vi "Read Fan Status.vi"(11 "Update Fan Status Msg in":refnum<class "Update Fan Status Msg.lvclass">) -> (1 "Fan B":T1, 2 "Fan A":T1)   [LabVIEW 2018, in "Dual Fan.lvlib" / "Update Fan Status Msg.lvclass"]
doc: "Reads the fan status recorded in this message."
uses:
  Update Fan Status Msg.lvclass
  Dual Fan/Fan Info.ctl
  Update Fan Status Msg.lvclass/Update Fan Status Msg.ctl
  Dual Fan/Dual Fan.lvclass
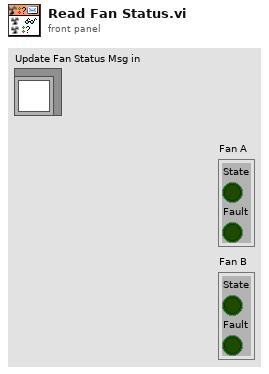
[diagram p1: front panel]
types:
  T1 = typedef "Dual Fan.lvlib/Dual Fan.lvclass/Fan Info.ctl" = cluster{"State":bool, "Fault":bool}
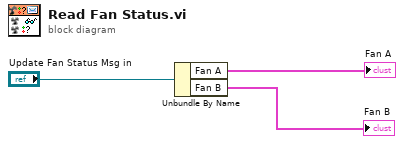
[diagram p0: block diagram]
diagram:
  n1 = Unbundle By Name("Update Fan Status Msg in") -> ("Fan A"=→"Fan A":T1, "Fan B"=→"Fan B":T1)
